vi "SingleAxisControl.vi"() -> ()   [LabVIEW 2013]
uses:
  Motion/HomeSingle.vi
  Motion/EnableSingle.vi
  Motion/FaultAckSingle.vi
  Motion/DisableSingle.vi
  Motion/AbortSingle.vi
  Motion/MoveIncSingle.vi
  Motion/FreerunSingle.vi
  Parameters/GetAxisParameterString.vi
  Parameters/GetAxisParameterDouble.vi
panel:
  in  "Abort":bool
  out "do stop":bool
  out "Vel Units":string
  out "Pos Units":string
  in  "stop":bool
  out "Vel Fbk":dbl
  out "Pos Fbk":dbl
  out "Status":string
  in  "Jog Right":bool
  in  "Jog Left":bool
  in  "Distance":dbl=1000.0 min=0.0 max=10.0
  in  "Speed":dbl=5000.0 min=0.0 max=50.0
  in  "Jog":bool
  in  "FaultAck":bool
  in  "Home":bool
  in  "Disable":bool
  in  "Enable":bool
  out "Axis":string
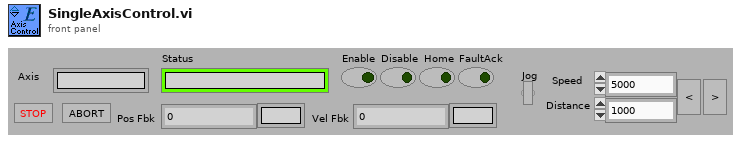
[diagram p1: front panel]
types:
  T1 = cluster{"new reference":refnum<k24>, "Event Callback":refnum<k27>, "ControllerDiagPacket":refnum<user-event>, "Event Registration Refnum":refnum<event-registration>}
  T2 = typedef "AxisDiagPacket.ctl" = cluster{"Axis Name":string, "Acceleration Command":dbl, "Amplifier Temperature":sgl, "Analog Input 0":dbl, "Analog Input 1":dbl, "Analog Output 0":dbl, "Analog Output 1":dbl, "Axis Fault (num)":i32, "Axis Fault (str)":string, "Axis Fault (bits)":cluster{"AmplifierFault":bool, "AmplifierTemperatureFault":bool, "CcwEndOfTravelLimitFault":bool, "CcwSoftwareLimitFault":bool, "CommunicationLostFault":bool, "CwEndOfTravelLimitFault":bool, "CwSoftwareLimitFault":bool, "EmergencyStopFault":bool, "EncoderFault":bool, "ExternalFault":bool, "FeedbackScalingFault":bool, "HallSensorFault":bool, "MarkerSearchFault":bool, "MaxVelocityCommandFault":bool, "MotorTemperatureFault":bool, "None":bool, "OverCurrentFault":bool, "PositionErrorFault":bool, "PositionFeedbackFault":bool, "VelocityErrorFault":bool, "VelocityFeedbackFault":bool, "VoltageClampFault":bool, "PowerSupplyFault":bool}, "Axis Status (num)":i32, "Axis Status (str)":string, "Axis Status (bits)":cluster{"AccelerationPhase":bool, "AutofocusActive":bool, "BrakeOutput":bool, "CalibrationActive":bool, "CalibrationEnabled":bool, "CcwEndOfTravelLimitInput":bool, "CommandShapingFilterDone":bool, "CosineEncoderError":bool, "CurrentClamp":bool, "CwEndOfTravelLimitInput":bool, "DecelerationPhase":bool, "EmergencyStopInput":bool, "Enabled":bool, "GantryMasterActive":bool, "GantryModeActive":bool, "HallAInput":bool, "HallBInput":bool, "HallCInput":bool, "Homed":bool, "HomeLimitInput":bool, "Homing":bool, "InPosition":bool, "InPosition2":bool, "JoystickControl":bool, "MarkerInput":bool, "MasterMotionSuppressed":bool, "MasterSlaveControl":bool, "MotionIsCw":bool, "MoveActive":bool, "None":bool, "PositionCaptureActive":bool, "ServoControl":bool, "SineEncoderError":bool}, "Current Command":sgl, "Current Error":sgl, "Current Feedback":sgl, "Digital Input 0":i32, "Digital Input 1":i32, "Digital Input 2":i32, "Digital Output 0":i32, "Digital Output 1":i32, "Digital Output 2":i32, "Position Feedback Auxiliary":dbl, "Position Command":dbl, "Position Error":dbl, "Position Feedback":dbl, "Program Position Command":dbl, "Program Position Error":dbl, "Program Position Feedback":dbl, "Velocity Command":dbl, "Velocity Error":dbl, "Velocity Feedback":dbl}
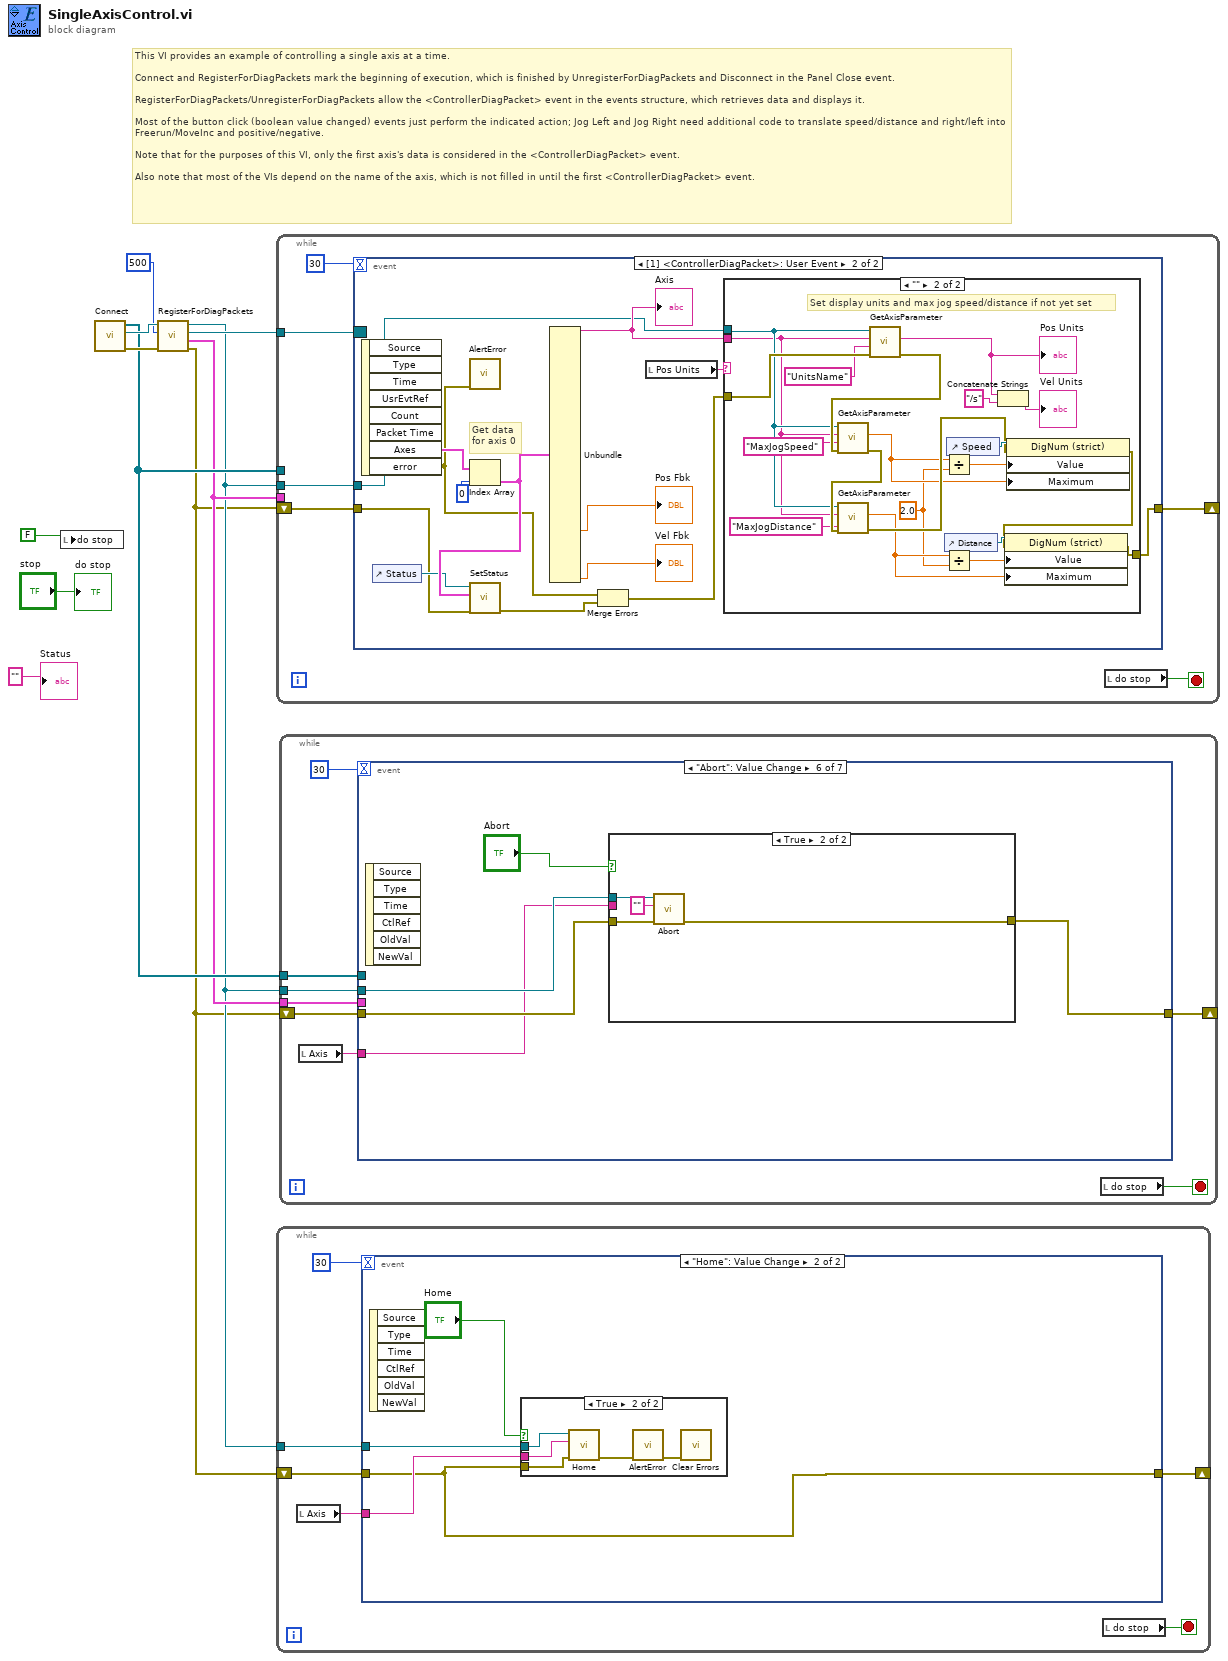
[diagram p0: block diagram]
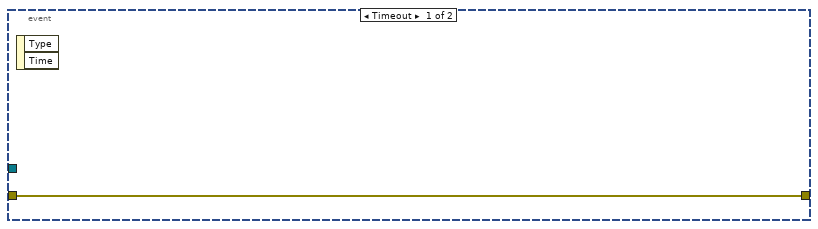
[diagram p2: hidden frame]
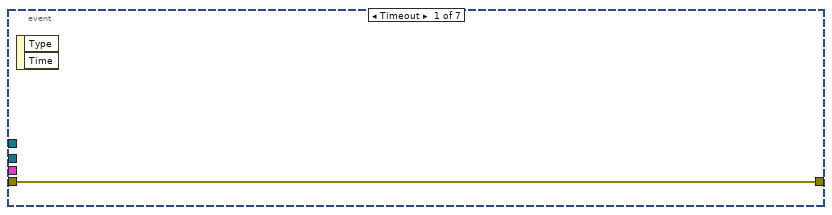
[diagram p4: hidden frame]
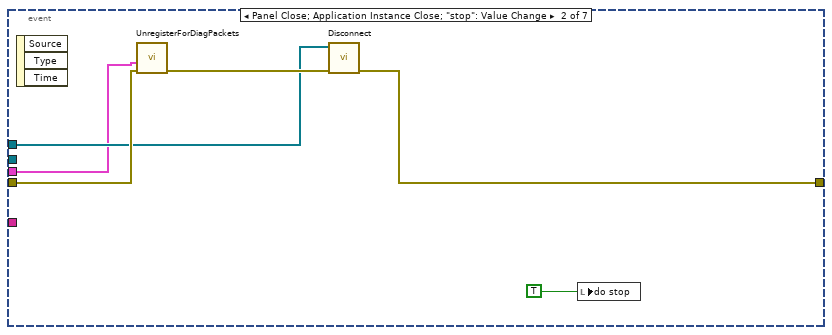
[diagram p5: hidden frame]
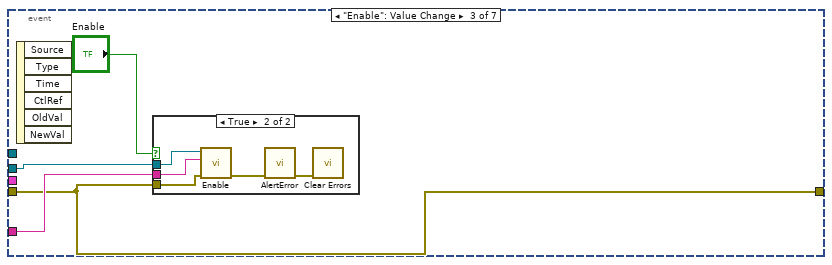
[diagram p6: hidden frame]
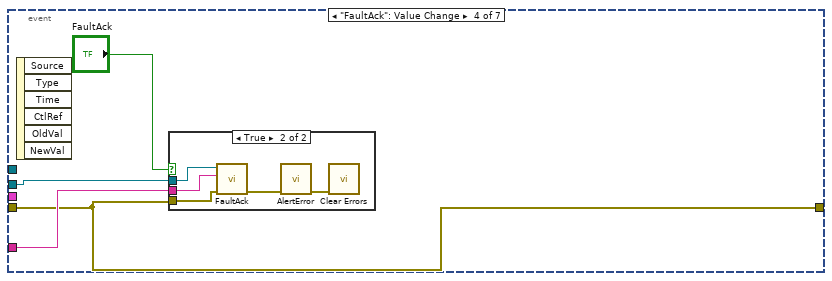
[diagram p8: hidden frame]
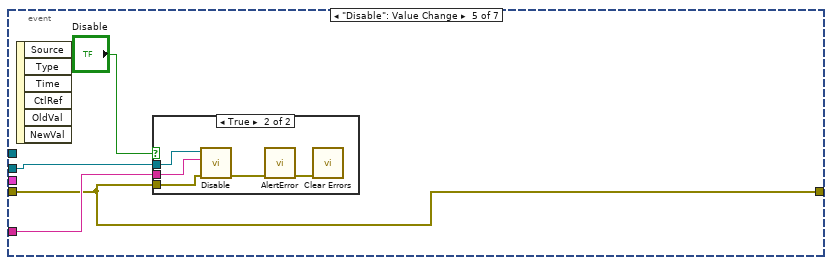
[diagram p10: hidden frame]
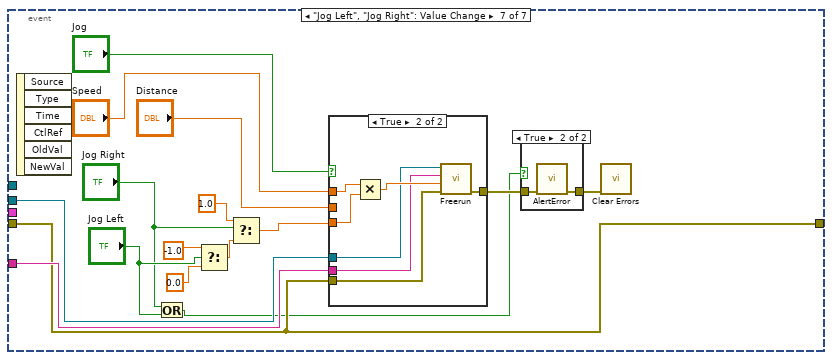
[diagram p13: hidden frame]
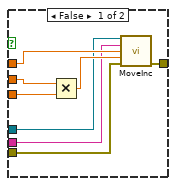
[diagram p15: hidden frame]
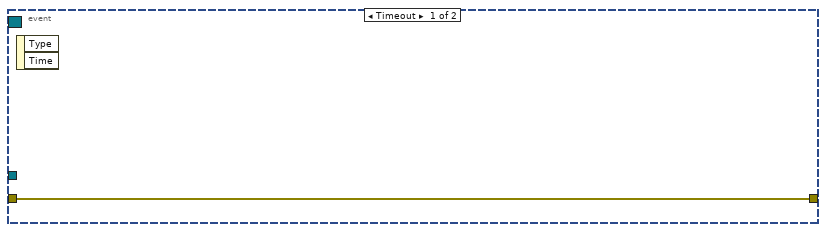
[diagram p16: hidden frame]
diagram:
  # "This VI provides an example of controlling a single axis at a time. \n\nConnect and RegisterForDiagPackets mark the beginning of execution, which is finished by UnregisterForDiagPackets and Disconnect in the Panel Close event.\n\nRegisterForDiagPackets/UnregisterForDiagPackets allow the <ControllerDiagPacket> event in the events structure, which retrieves data and displays it.\n\nMost of the button click (boolean value changed) events just perform the indicated action; Jog Left and Jog Right need additional code to translate speed/distance and right/left into Freerun/MoveInc and positive/negative.\n\nNote that for the purposes of this VI, only the first axis's data is considered in the <ControllerDiagPacket> event.\n\nAlso note that most of the VIs depend on the name of the axis, which is not filled in until the first <ControllerDiagPacket> event."
  n1 = local write "do stop"(FALSE ("do stop")) -> ()
  n2 = call "Connect.vi"() -> ("error out"=w8:errorcluster, "controller"=w9:refnum<k24>, "controllers"=w7:refnum<k24>[])  [unwired: 9 in]
  n3 = call "RegisterForDiagPackets.vi"("error in (no error)"=w8, "refresh interval (default)"=500, "Controller in"=w9) -> ("error out"=w4:errorcluster, "Even Metadata"=w6:T1, "Event Registration Refnum"=w11:refnum<event-registration>, "Controller out"=w5:refnum<k24>)  [unwired: 4 in]
  n4 = while {
    tunnel: w11 -> [w16]
    tunnel: w6 -> [_]
    tunnel: w5 -> [w15]
    shift-right: [w13] -> _
    shift-left: w4 -> [w14]
    tunnel: w7 -> [_]
    stop <- w12 stop-if-true
    n5 = event shown="[1] <ControllerDiagPacket>: User Event" {
      selector: w16 -> [_ _]
      dyn-events: _ -> [_ _]
      timeout: 30 -> [_ _]
      tunnel: w15 -> [_ w21]
      tunnel: w14 -> [w18 w20]
      tunnel: [w18 w19] -> w13
      event Timeout {
        n6 = event-data() -> ()  [unwired: 1 in, 2 out]
      }
      event User Event {
        # "Get data for axis 0"
        n7 = event-data() -> ("Axes"=w23:T2[], "error"=w22:errorcluster)  [unwired: 1 in, 6 out]
        n8 = control-ref of="Status"() -> (w25:refnum<vi>)
        n9 = call "AlertError.vi"("error in (no error)"=w22) -> ()  [unwired: 10 in, 1 out]
        n10 = Index Array(array=w23, index=0) -> (element=w26:T2)
        n11 = call "SetStatus.vi"("error in (no error)"=w20, "AxisDiagPacket"=w26, "Status string"=w25) -> ("error out"=w27:errorcluster)  [unwired: 8 in]
        n12 = Unbundle(w26) -> ("Axis Name"=w30:string, "Position Feedback"=→"Pos Fbk":dbl, "Velocity Feedback"=→"Vel Fbk":dbl)  [unwired: 29 out]
        "Axis" <- w30
        n13 = Merge Errors(w22, w27) -> (w31:errorcluster)
        n14 = local read "Pos Units"() -> (w32:string)
        n15 = case shown="\"\"" w32 {
          tunnel: w30 -> [_ w46]
          tunnel: w21 -> [_ w47]
          tunnel: w31 -> [w33 w51]
          tunnel: [w33 w41] -> w19
          frame Default {
          }
          frame "" {
            w34 = 2.0 ("y")
            # "Set display units and max jog speed/distance if not yet set"
            n16 = call-poly "GetAxisParameter.vi"("error in (no error)"=w51, "Parameter Name"="UnitsName" ("parameter name"), "axis name"=w46, "controller in"=w47) -> ("error out"=w48:errorcluster, "value"=w52:string)  [unwired: 5 in, 1 out]
            "Pos Units" <- w52
            n17 = call-poly "GetAxisParameter.vi"("error in (no error)"=w48, "Parameter Name"="MaxJogSpeed" ("parameter name"), "axis name"=w46, "controller in"=w47) -> ("error out"=w49:errorcluster, "value"=w36:dbl)  [unwired: 5 in, 1 out]
            n18 = call-poly "GetAxisParameter.vi"("error in (no error)"=w49, "Parameter Name"="MaxJogDistance" ("parameter name"), "axis name"=w46, "controller in"=w47) -> ("error out"=w39:errorcluster, "value"=w35:dbl)  [unwired: 5 in, 1 out]
            n19 = Divide(x=w36, y=w34) -> (x/y=w37:dbl)
            n20 = Divide(x=w35, y=w34) -> (x/y=w38:dbl)
            n21 = control-ref of="Distance"() -> (w42:refnum<vi>)
            n22 = control-ref of="Speed"() -> (w43:refnum<vi>)
            n23 = Concatenate Strings(w52, "/s" ("string")) -> (→"Vel Units":string)
            n24 = property class="DigNum (strict)"(reference=w43, error in=w39, "Value"=w37, "Maximum"=w36) -> (error out=w40:errorcluster)  [unwired: 1 out]
            n25 = property class="DigNum (strict)"(reference=w42, error in=w40, "Value"=w38, "Maximum"=w35) -> (error out=w41:errorcluster)  [unwired: 1 out]
          }
        }
      }
    }
    n26 = local read "do stop"() -> (w12:bool)
  }
  n27 = while {
    tunnel: w5 -> [w58]
    shift-right: [w55] -> _
    shift-left: w4 -> [w57]
    stop <- w60 stop-if-true
    n28 = local read "Axis"() -> (w56:string)
    n29 = event shown="[1] \"Home\": Value Change" {
      selector: _ -> [_ _]
      dyn-events: _ -> [_ _]
      timeout: 30 -> [_ _]
      tunnel: w58 -> [_ w64]
      tunnel: w57 -> [w61 w62]
      tunnel: w56 -> [_ w63]
      tunnel: [w61 w62] -> w55
      event Timeout {
        n30 = event-data() -> ()  [unwired: 1 in, 2 out]
      }
      event "Home": Value Change {
        n31 = event-data() -> ()  [unwired: 1 in, 6 out]
        n32 = case shown="True" "Home" {
          tunnel: w64 -> [_ w70]
          tunnel: w62 -> [_ w68]
          tunnel: w63 -> [_ w69]
          frame False {
          }
          frame True {
            n33 = call-poly "Home.vi"("error in (no error)"=w68, "axis name"=w69, "controller in"=w70) -> ("error out"=w67:errorcluster)  [unwired: 7 in, 1 out]
            n34 = call "AlertError.vi"("error in (no error)"=w67) -> ("error out"=w66:errorcluster)  [unwired: 10 in]
            n35 = call <vilib>:"Clear Errors.vi"("error in (no error)"=w66) -> ()  [unwired: 6 in, 1 out]
          }
        }
      }
    }
    n36 = local read "do stop"() -> (w60:bool)
  }
  n37 = while {
    tunnel: w7 -> [w78]
    tunnel: w6 -> [w76]
    tunnel: w5 -> [w75]
    shift-right: [w71] -> _
    shift-left: w4 -> [w77]
    stop <- w72 stop-if-true
    n38 = local read "Axis"() -> (w74:string)
    n39 = event shown="[5] \"Abort\": Value Change" {
      selector: _ -> [_ _ _ _ _ _ _]
      dyn-events: _ -> [_ _ _ _ _ _ _]
      timeout: 30 -> [_ _ _ _ _ _ _]
      tunnel: w76 -> [_ w80 _ _ _ _ _]
      tunnel: w75 -> [_ _ w89 w98 w106 w115 w129]
      tunnel: w77 -> [w79 w85 w86 w96 w104 w116 w128]
      tunnel: [w79 w83 w86 w96 w104 w114 w128] -> w71
      tunnel: w74 -> [_ _ w88 w97 w105 w113 w130]
      tunnel: w78 -> [_ w82 _ _ _ _ _]
      event Timeout {
        n40 = event-data() -> ()  [unwired: 1 in, 2 out]
      }
      event Panel Close; Application Instance Close; "stop": Value Change {
        n41 = event-data() -> ()  [unwired: 1 in, 3 out]
        n42 = call "UnregisterForDiagPackets.vi"("error in (no error)"=w85, "Even Metadata"=w80) -> ("error out"=w84:errorcluster)  [unwired: 9 in]
        n43 = call "Disconnect.vi"("error in (no error)"=w84, "controllers"=w82) -> ("error out"=w83:errorcluster)  [unwired: 9 in]
        n44 = local write "do stop"(TRUE) -> ()
      }
      event "Enable": Value Change {
        n45 = event-data() -> ()  [unwired: 1 in, 6 out]
        n46 = case shown="True" "Enable" {
          tunnel: w89 -> [_ w93]
          tunnel: w86 -> [_ w91]
          tunnel: w88 -> [_ w92]
          frame False {
          }
          frame True {
            n47 = call-poly "Enable.vi"("error in (no error)"=w91, "axis name"=w92, "controller in"=w93) -> ("error out"=w90:errorcluster)  [unwired: 7 in, 1 out]
            n48 = call "AlertError.vi"("error in (no error)"=w90) -> ("error out"=w94:errorcluster)  [unwired: 10 in]
            n49 = call <vilib>:"Clear Errors.vi"("error in (no error)"=w94) -> ()  [unwired: 6 in, 1 out]
          }
        }
      }
      event "FaultAck": Value Change {
        n50 = event-data() -> ()  [unwired: 1 in, 6 out]
        n51 = case shown="True" "FaultAck" {
          tunnel: w98 -> [_ w103]
          tunnel: w96 -> [_ w101]
          tunnel: w97 -> [_ w102]
          frame False {
          }
          frame True {
            n52 = call-poly "FaultAck.vi"("error in (no error)"=w101, "axis name"=w102, "controller in"=w103) -> ("error out"=w100:errorcluster)  [unwired: 7 in, 1 out]
            n53 = call "AlertError.vi"("error in (no error)"=w100) -> ("error out"=w99:errorcluster)  [unwired: 10 in]
            n54 = call <vilib>:"Clear Errors.vi"("error in (no error)"=w99) -> ()  [unwired: 6 in, 1 out]
          }
        }
      }
      event "Disable": Value Change {
        n55 = event-data() -> ()  [unwired: 1 in, 6 out]
        n56 = case shown="True" "Disable" {
          tunnel: w106 -> [_ w112]
          tunnel: w104 -> [_ w110]
          tunnel: w105 -> [_ w111]
          frame False {
          }
          frame True {
            n57 = call-poly "Disable.vi"("error in (no error)"=w110, "axis name"=w111, "controller in"=w112) -> ("error out"=w109:errorcluster)  [unwired: 7 in, 1 out]
            n58 = call "AlertError.vi"("error in (no error)"=w109) -> ("error out"=w108:errorcluster)  [unwired: 10 in]
            n59 = call <vilib>:"Clear Errors.vi"("error in (no error)"=w108) -> ()  [unwired: 6 in, 1 out]
          }
        }
      }
      event "Abort": Value Change {
        n60 = event-data() -> ()  [unwired: 1 in, 6 out]
        n61 = case shown="True" "Abort" {
          tunnel: w115 -> [_ w122]
          tunnel: w116 -> [w118 w121]
          tunnel: [w118 w120] -> w114
          tunnel: w113 -> [_ _]
          frame False {
          }
          frame True {
            n62 = call-poly "Abort.vi"("error in (no error)"=w121, "axis name? (all)"="", "controller in"=w122) -> ("error out"=w120:errorcluster)  [unwired: 7 in, 1 out]
          }
        }
      }
      event "Jog Left", "Jog Right": Value Change {
        n63 = event-data() -> ()  [unwired: 1 in, 6 out]
        n64 = Or(x="Jog Right", y="Jog Left") -> (x .or. y?=w123:bool)
        n65 = Select(t=-1.0, s="Jog Left", f=0.0) -> (s? t:f=w138:dbl)
        n66 = Select(t=1.0, s="Jog Right", f=w138) -> (s? t:f=w134:dbl)
        n67 = case shown="True" "Jog" {
          tunnel: "Speed" -> [w144 w156]
          tunnel: "Distance" -> [w149 _]
          tunnel: w134 -> [w148 w155]
          tunnel: w128 -> [w147 w154]
          tunnel: w130 -> [w143 w152]
          tunnel: w129 -> [w142 w151]
          tunnel: [w146 w150] -> w126
          frame False {
            n68 = Multiply(x=w149, y=w148) -> (x*y=w145:dbl)
            n69 = call-poly "MoveInc.vi"("controller in"=w142, "axis name"=w143, "speed"=w144, "distance"=w145, "error in (no error)"=w147) -> ("error out"=w146:errorcluster)  [unwired: 9 in, 1 out]
          }
          frame True {
            n70 = Multiply(x=w156, y=w155) -> (x*y=w153:dbl)
            n71 = call-poly "Freerun.vi"("error in (no error)"=w154, "speed"=w153, "axis name"=w152, "controller in"=w151) -> ("error out"=w150:errorcluster)  [unwired: 6 in, 1 out]
          }
        }
        n72 = case shown="True" w123 {
          tunnel: [w139 w141] -> w127
          tunnel: w126 -> [w139 w140]
          frame False {
          }
          frame True {
            n73 = call "AlertError.vi"("error in (no error)"=w140) -> ("error out"=w141:errorcluster)  [unwired: 10 in]
          }
        }
        n74 = call <vilib>:"Clear Errors.vi"("error in (no error)"=w127) -> ()  [unwired: 6 in, 1 out]
      }
    }
    n75 = local read "do stop"() -> (w72:bool)
  }
  "Status" <- "" ("Status")
  "do stop" <- "stop"
